vi "AddPassed.vi"(8 "error in (no error)":errorcluster, 10 "TestCase":refnum<class "TestCase.lvclass">, 11 "ResultTreeListener in":refnum<class "ResultTreeListener.lvclass">) -> (0 "error out":errorcluster, 3 "ResultTreeListener out":refnum<class "ResultTreeListener.lvclass">)   [LabVIEW 2019, in "ResultTreeListener.lvclass"]
doc: "A test passed."
uses:
  ResultTreeListener.lvclass
  TestCase/TestCase/TestCase.lvclass
  ResultTree/Icon.ctl
  ResultTree/ResultTree.lvclass
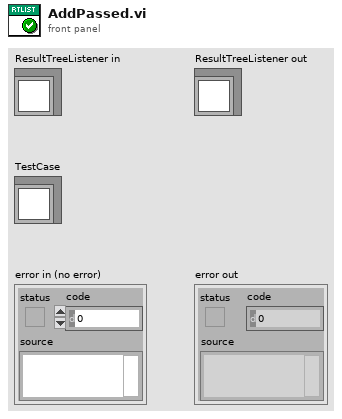
[diagram p1: front panel]
types:
  T1 = typedef "ResultTree.lvclass/Icon.ctl" = enum16{"None", "Passed", "Failed", "Error"}
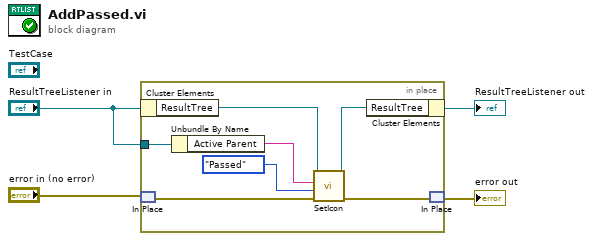
[diagram p0: block diagram]
diagram:
  n1 = in-place {
    in-place-border: "ResultTreeListener in" -> [w10]
    n2 = in-place-cluster #1("ResultTreeListener in") -> ("ResultTree"=w11:refnum<class "ResultTree.lvclass">)
    n3 = in-place-match #2("error in (no error)") -> (w8:errorcluster)
    n4 = Unbundle By Name(w10) -> ("Active Parent"=w7:string)
    n5 = call "SetIcon.vi"("error in (no error)"=w8, "Icon"=Icon."Passed", "Tag Name"=w7, "ResultTree in"=w11) -> ("error out"=w5:errorcluster, "ResultTree out"=w6:refnum<class "ResultTree.lvclass">)  [unwired: 6 in]
    n6 = in-place-cluster #1("ResultTree"=w6) -> (→"ResultTreeListener out":refnum<class "ResultTreeListener.lvclass">)
    n7 = in-place-match #2(w5) -> (→"error out":errorcluster)
  }
